vi "Change Temperature.vi"(8 "error in (no error)":errorcluster, 11 "Test Framework in":refnum<class "Test Framework.lvclass">) -> (0 "error out":errorcluster, 1 "Soak Time Used":dbl, 2 "User Aborted":bool, 3 "Test Framework out":refnum<class "Test Framework.lvclass">)   [LabVIEW 2020, in "Test Framework.lvclass"]
uses:
  Test Framework.lvclass
  Instruments/Temperature Control/Controls/Set point.ctl
  Test Framework.lvclass/Test Framework.ctl
  Instruments/Temperature Control/Temperature Control.lvclass/Temperature Control.ctl
  Instruments/Temperature Control/Controls/Head and Air actions.ctl
  Instruments/Temperature Control/Temperature Control.lvclass
panel:
  out "Set Point":T1
  out "Set Temperature [degC]":dbl
  out "Current Temperature [degC]":dbl
  in  "Skip Soak Button":bool
  in  "Abort Button":bool
  out "Remaning Soak Time":string
  out "Elapsed Time":string
  out "Temp Graph":cluster{"X":dbl, "Y":dbl}[](graph)
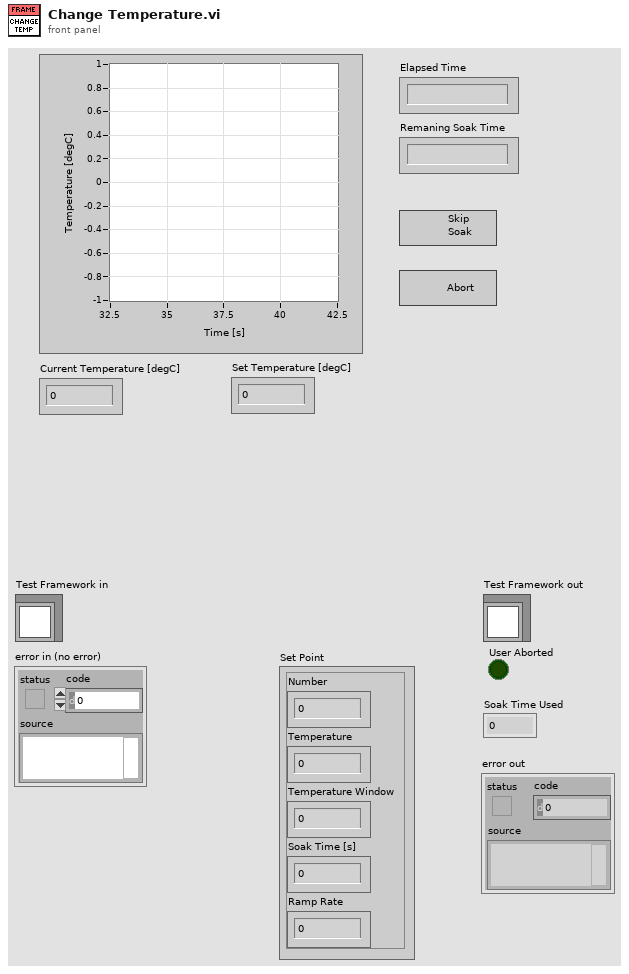
[diagram p1: front panel]
types:
  T1 = typedef "Temperature Control.lvclass/Set point.ctl" = cluster{"Number":u32, "Temperature":dbl, "Temperature Window":dbl, "Soak Time [s]":u32, "Ramp Rate":dbl}
  T2 = enum8{"Enabled", "Disabled", "Disabled and Grayed Out"}
  T3 = enum16{"Query Temp", "Update Graph", "Start Soak", "Done", "Abort", "Skip Soak"}
  T4 = typedef "Temperature Control.lvclass/Head and Air actions.ctl" = enum16{"Head Down & Air On", "Head Up & Air Off", "Head Down", "Head Up", "Air On", "Air Off", "Compressor On", "Compressor Off"}
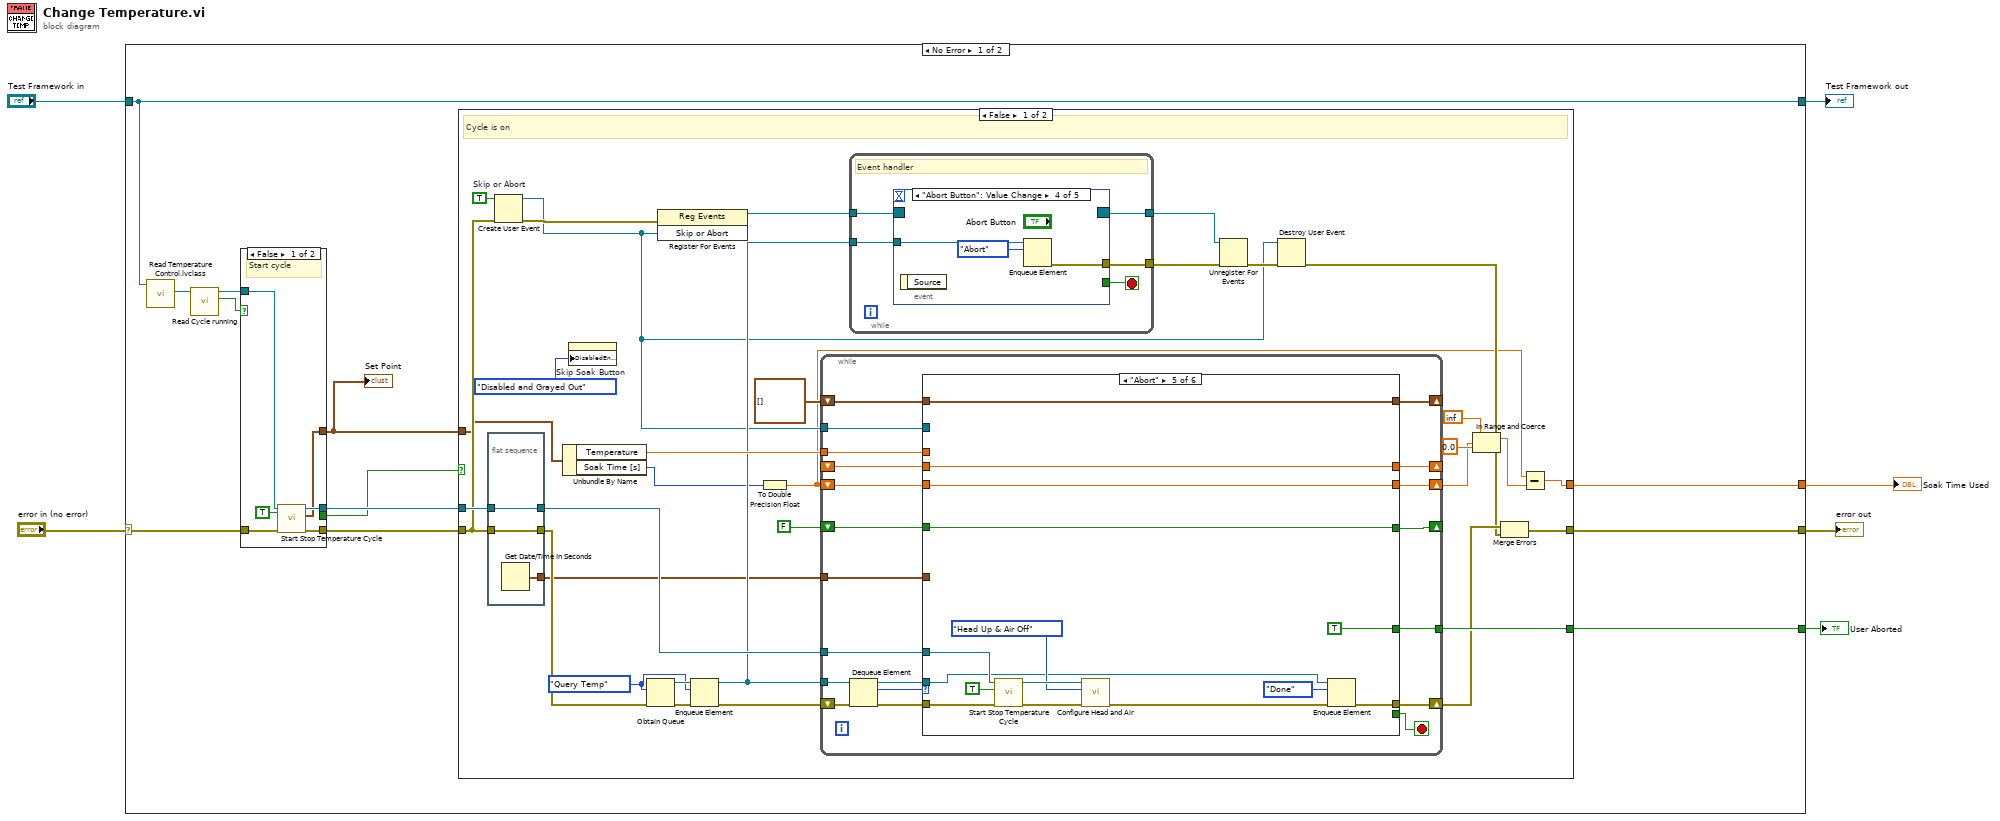
[diagram p0: block diagram]
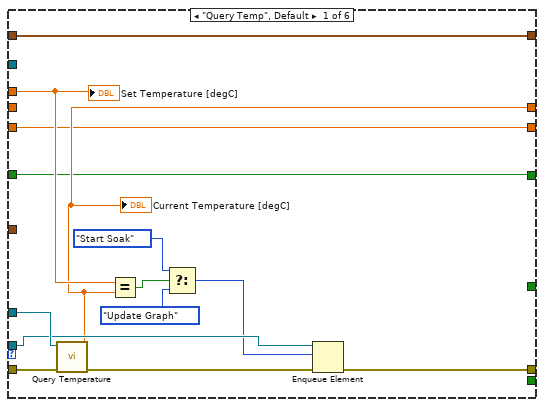
[diagram p2: hidden frame]
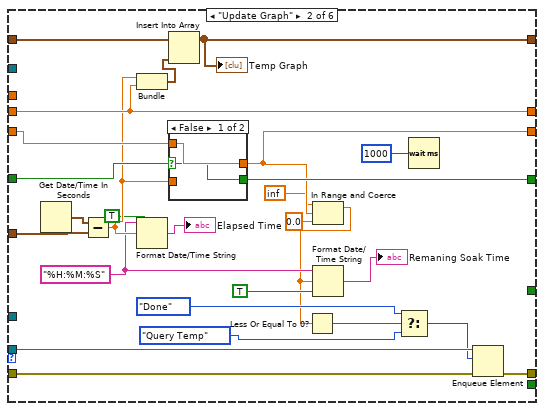
[diagram p3: hidden frame]
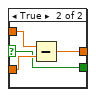
[diagram p4: hidden frame]
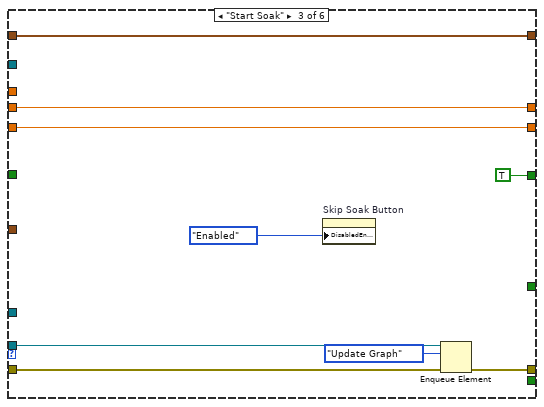
[diagram p5: hidden frame]
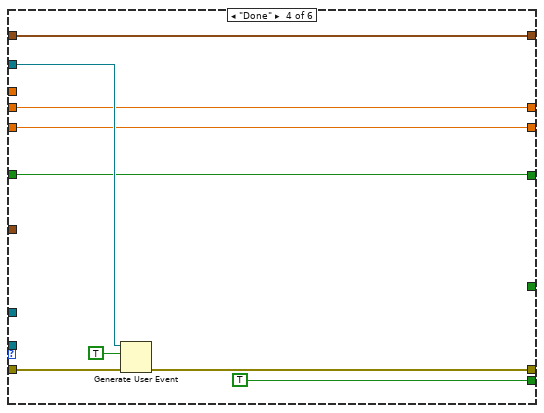
[diagram p6: hidden frame]
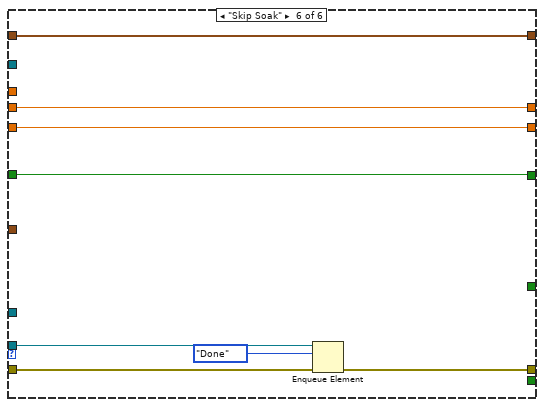
[diagram p7: hidden frame]
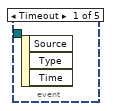
[diagram p8: hidden frame]
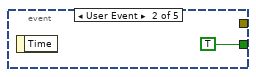
[diagram p9: hidden frame]
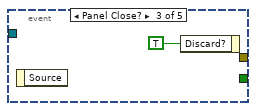
[diagram p10: hidden frame]
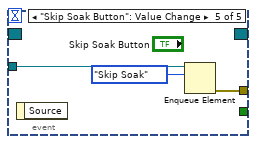
[diagram p11: hidden frame]
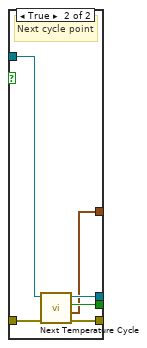
[diagram p13: hidden frame]
diagram:
  n1 = case shown="No Error" "error in (no error)" {
    selector: "error in (no error)" -> [w15 w190]
    tunnel: [w10 w190] -> w5
    tunnel: [w7 w189] -> w3
    tunnel: "Test Framework in" -> [w7 w189]
    tunnel: [w11 _] -> w2
    tunnel: [w9 _] -> w1
    frame No Error {
      n2 = call "Read Temperature Control.lvclass.vi"("Test Framework in"=w7) -> ("Temperature Control.lvclass"=w18:refnum<class "Temperature Control.lvclass">)  [unwired: 9 in, 1 out]
      n3 = call "Read Cycle running.vi"("Temperature Control in"=w18) -> ("Cycle running"=w17:bool, "Temperature Control out"=w16:refnum<class "Temperature Control.lvclass">)  [unwired: 9 in]
      n4 = case shown="False" w17 {
        tunnel: w16 -> [w182 w187]
        tunnel: w15 -> [w180 w188]
        tunnel: [_ w186] -> w12
        tunnel: [w179 w185] -> w13
        tunnel: [w178 w184] -> w14
        tunnel: [w177 w183] -> w8
        frame False {
          # "Start cycle"
          n5 = call-dynamic "Start Stop Temperature Cycle.vi"("error in (no error)"=w180, "Start/Stop Cycle"=TRUE, "Temperature Control in"=w182) -> ("error out"=w179:errorcluster, "Set Point"=w177:T1, "Temperature Control out"=w178:refnum<class "Temperature Control.lvclass">)  [unwired: 6 in]
        }
        frame True {
          # "Next cycle point"
          n6 = call-dynamic "Next Temperature Cycle.vi"("error in (no error)"=w188, "Temperature Control in"=w187) -> ("error out"=w185:errorcluster, "Set Point"=w183:T1, "Temperature Finished"=w186:bool, "Temperature Control out"=w184:refnum<class "Temperature Control.lvclass">)  [unwired: 6 in]
        }
      }
      "Set Point" <- w8
      n7 = case shown="False" w12 {
        tunnel: w14 -> [w51 _]
        tunnel: w13 -> [w49 w176]
        tunnel: [w35 _] -> w11
        tunnel: [w28 w176] -> w10
        tunnel: [w24 _] -> w9
        tunnel: w8 -> [w19 _]
        frame False {
          w42 = T3."Query Temp" ("Change Temp state machine")
          w26 = TRUE  # Skip or Abort
          # "Cycle is on"
          n8 = flat-sequence {
            tunnel: w49 -> [w161]
            tunnel: w51 -> [w160]
            tunnel: [w161] -> w47
            tunnel: [w160] -> w45
            tunnel: [w162] -> w39
            frame #0 {
              n9 = Get Date/Time In Seconds() -> (seconds since 1Jan1904=w162:timestamp)
            }
          }
          n10 = Create User Event(user event datatype=w26, error in=w49) -> (user event=w29:refnum<user-event>, error out=w50:errorcluster)
          n11 = Unbundle By Name(w19) -> ("Temperature"=w46:dbl, "Soak Time [s]"=w37:u32)
          n12 = property on="Skip Soak Button" class="Bool"("DisabledEnum"=T2."Disabled and Grayed Out" ("Disabled")) -> ()  [unwired: 2 in, 2 out]
          n13 = Obtain Queue(element data type=w42, error in (no error)=w47) -> (queue out=w43:refnum<queue>, error out=w44:errorcluster)  [unwired: 3 in, 1 out]
          n14 = register-events(error in=w50, w29) -> (reference out=w48:refnum<event-registration>)  [unwired: 1 in, 1 out]
          n15 = Enqueue Element(queue=w43, element=w42, error in (no error)=w44) -> (queue out=w41:refnum<queue>, error out=w40:errorcluster)  [unwired: 1 in, 1 out]
          n16 = To Double Precision Float(number=w37) -> (double precision float=w25:dbl)
          n17 = while {
            tunnel: w41 -> [w68]
            tunnel: w39 -> [w71]
            tunnel: w46 -> [w70]
            tunnel: w29 -> [w64]
            shift-right: [w62] -> w34
            shift-left: w40 -> [w69]
            tunnel: w45 -> [w61]
            shift-right: [w59] -> _
            shift-left: cluster{"X":dbl, "Y":dbl}[] [] ("Temp Graph") -> [w60]
            shift-right: [w58] -> _
            shift-left: _ -> [w57]
            shift-right: [w53] -> w21
            shift-left: w25 -> [w56]
            shift-right: [w54] -> _
            shift-left: FALSE -> [w55]
            tunnel: [w52] -> w35
            stop <- w63 stop-if-true
            n18 = Dequeue Element(queue=w68, error in (no error)=w69) -> (queue out=w65:refnum<queue>, element=w67:T3, error out=w66:errorcluster)  [unwired: 1 in, 1 out]
            n19 = case shown="\"Abort\"" w67 {
              tunnel: w71 -> [_ w111 _ _ _ _]
              tunnel: w70 -> [w76 _ _ _ _ _]
              tunnel: w66 -> [w85 w96 w125 w136 w147 w155]
              tunnel: w65 -> [w80 w97 w124 _ w140 w154]
              tunnel: w64 -> [_ _ _ w135 _ _]
              tunnel: [w82 w98 w126 w133 w141 w153] -> w62
              tunnel: [_ _ _ TRUE _ _] -> w63
              tunnel: w61 -> [w84 _ _ _ w146 _]
              tunnel: w60 -> [w75 w109 w122 w128 w151 w159]
              tunnel: [w75 w107 w122 w128 w151 w159] -> w59
              tunnel: [w74 w106 w121 w129 w150 w158] -> w58
              tunnel: w57 -> [_ w106 w121 w129 w150 w158]
              tunnel: w56 -> [w73 w104 w120 w130 w149 w157]
              tunnel: w55 -> [w72 w105 _ w131 w148 w156]
              tunnel: [w72 w102 TRUE w131 w148 w156] -> w54
              tunnel: [w73 w89 w120 w130 w149 w157] -> w53
              tunnel: [_ _ _ _ TRUE _] -> w52
              frame "Query Temp", Default {
                n20 = call-dynamic "Query Temperature.vi"("error in (no error)"=w85, "Temperature Control in"=w84) -> ("error out"=w81:errorcluster, "Current Temperature [deg C]"=w74:dbl)  [unwired: 7 in, 1 out]
                "Current Temperature [degC]" <- w74
                n21 = Equal?(x=w76, y=w74) -> (x = y?=w83:bool)
                n22 = Select(t=T3."Start Soak" ("element"), s=w83, f=T3."Update Graph" ("element")) -> (s? t:f=w77:T3)
                n23 = Enqueue Element(queue=w80, element=w77, error in (no error)=w81) -> (error out=w82:errorcluster)  [unwired: 1 in, 2 out]
                "Set Temperature [degC]" <- w76
              }
              frame "Update Graph" {
                w101 = "%H:%M:%S" ("time format string (%c)")
                n24 = Get Date/Time In Seconds() -> (seconds since 1Jan1904=w112:timestamp)
                n25 = Subtract(x=w112, y=w111) -> (x-y=w103:dbl)
                n26 = Bundle(w103, "Current Temperature [deg C]"=w106) -> (w108:cluster{dbl, "Current Temperature [deg C]":dbl})  [unwired: 1 in]
                n27 = Format Date/Time String(time format string (%c)=w101, seconds (now)=w103, UTC format=TRUE) -> (date/time string=→"Elapsed Time":string)
                n28 = Insert Into Array(array=w109, new element=w108) -> (w107:cluster{"X":dbl, "Y":dbl}[])  [unwired: 1 in]
                "Temp Graph" <- w107
                n29 = case shown="False" w105 {
                  selector: w105 -> [w113 w115]
                  tunnel: w104 -> [w114 w118]
                  tunnel: w103 -> [_ w117]
                  tunnel: [w114 w116] -> w89
                  tunnel: [w113 w115] -> w102
                  frame False {
                  }
                  frame True {
                    n30 = Subtract(x=w118, y=w117) -> (x-y=w116:dbl)
                  }
                }
                n31 = In Range and Coerce(upper limit=inf, x=w89, lower limit=0.0) -> (coerced(x)=w88:dbl)  [unwired: 1 out]
                n32 = Less Or Equal To 0?(x=w88) -> (x <= 0?=w99:bool)
                n33 = Format Date/Time String(time format string (%c)=w101, seconds (now)=w88, UTC format=TRUE) -> (date/time string=→"Remaning Soak Time":string)
                n34 = Select(t=T3."Done" ("Change Temp state machine"), s=w99, f=T3."Query Temp" ("Change Temp state machine")) -> (s? t:f=w95:T3)
                n35 = Wait (ms)(milliseconds to wait=u32 1000) -> ()  [unwired: 1 out]
                n36 = Enqueue Element(queue=w97, element=w95, error in (no error)=w96) -> (error out=w98:errorcluster)  [unwired: 1 in, 2 out]
              }
              frame "Start Soak" {
                n37 = property on="Skip Soak Button" class="Bool"("DisabledEnum"=T2."Enabled" ("Disabled")) -> ()  [unwired: 2 in, 2 out]
                n38 = Enqueue Element(queue=w124, element=T3."Update Graph", error in (no error)=w125) -> (error out=w126:errorcluster)  [unwired: 1 in, 2 out]
              }
              frame "Done" {
                n39 = Generate User Event(user event=w135, event data cluster=TRUE ("event data"), error in=w136) -> (error out=w133:errorcluster)  [unwired: 1 in, 1 out]
              }
              frame "Abort" {
                n40 = call-dynamic "Start Stop Temperature Cycle.vi"("error in (no error)"=w147, "Start/Stop Cycle"=TRUE, "Temperature Control in"=w146) -> ("error out"=w144:errorcluster, "Temperature Control out"=w143:refnum<class "Temperature Control.lvclass">)  [unwired: 6 in, 1 out]
                n41 = call-dynamic "Configure Head and Air.vi"("error in (no error)"=w144, "Head and Air actions"=Head_and_Air_actions."Head Up & Air Off", "Temperature Control in"=w143) -> ("error out"=w139:errorcluster)  [unwired: 7 in, 1 out]
                n42 = Enqueue Element(queue=w140, element=T3."Done", error in (no error)=w139) -> (error out=w141:errorcluster)  [unwired: 1 in, 2 out]
              }
              frame "Skip Soak" {
                n43 = Enqueue Element(queue=w154, element=T3."Done", error in (no error)=w155) -> (error out=w153:errorcluster)  [unwired: 1 in, 2 out]
              }
            }
          }
          n44 = while {
            tunnel: w48 -> [w167]
            tunnel: w41 -> [w165]
            tunnel: [w164] -> w31
            tunnel: [w163] -> w32
            stop <- w166 stop-if-true
            # "Event handler"
            n45 = event shown="[3] \"Abort Button\": Value Change" {
              selector: w167 -> [_ _ _ _ _]
              dyn-events: [_ _ _ _ _] -> w163
              timeout: _ -> [_ _ _ _ _]
              tunnel: [_ TRUE _ _ _] -> w166
              tunnel: w165 -> [_ _ _ w172 w174]
              tunnel: [_ _ _ w171 w175] -> w164
              event Timeout {
                n46 = event-data() -> ()  [unwired: 1 in, 3 out]
              }
              event User Event {
                n47 = event-data() -> ()  [unwired: 1 in, 1 out]
              }
              event Panel Close? {
                n48 = event-data() -> ()  [unwired: 1 in, 1 out]
                n49 = event-data("Discard?"=TRUE) -> ()  [unwired: 1 in, 1 out]
              }
              event "Abort Button": Value Change {
                n50 = event-data() -> ()  [unwired: 1 in, 1 out]
                n51 = Enqueue Element(queue=w172, element=T3."Abort") -> (error out=w171:errorcluster)  [unwired: 2 in, 2 out]
              }
              event "Skip Soak Button": Value Change {
                n52 = event-data() -> ()  [unwired: 1 in, 1 out]
                n53 = Enqueue Element(queue=w174, element=T3."Skip Soak") -> (error out=w175:errorcluster)  [unwired: 2 in, 2 out]
              }
            }
          }
          n54 = Unregister For Events(event registration refnum=w32, error in=w31) -> (error out=w30:errorcluster)
          n55 = Destroy User Event(user event=w29, error in=w30) -> (error out=w27:errorcluster)
          n56 = In Range and Coerce(upper limit=inf, x=w21, lower limit=0.0) -> (coerced(x)=w20:dbl)  [unwired: 1 out]
          n57 = Merge Errors(w34, w27) -> (w28:errorcluster)
          n58 = Subtract(x=w25, y=w20) -> (x-y=w24:dbl)
        }
        frame True {
          # "Cycling done"
        }
      }
    }
    frame Error {
    }
  }
  "error out" <- w5
  "Test Framework out" <- w3
  "User Aborted" <- w2
  "Soak Time Used" <- w1
